vi "读取.vi"() -> ()   [LabVIEW 2018]
uses:
  <vilib>/Utility/file.llb/Read Delimited Spreadsheet (string).vi
panel:
  out "all rows":string[][](array[string]) caption="所有行"
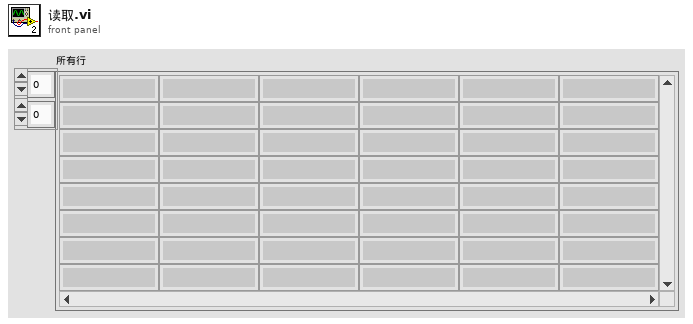
[diagram p1: front panel]
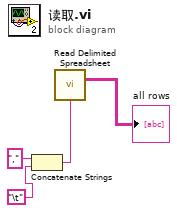
[diagram p0: block diagram]
diagram:
  n1 = Concatenate Strings("," ("字符串"), "\t") -> (w1:string)
  n2 = call-poly <vilib>:"Read Delimited Spreadsheet.vi"("delimiter (\\t)"=w1) -> ("all rows"=→"all rows":string[][])  [unwired: 9 in, 5 out]
